vi "ProcessFMData.vi"(1 "Sensor Readings In":dbl[](array[numeric])) -> (0 "Sensor Readings Out":dbl[](array[numeric]))   [LabVIEW 2018]
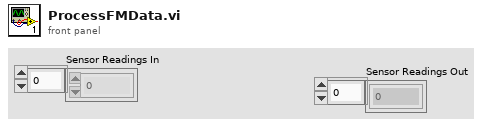
[diagram p1: front panel]
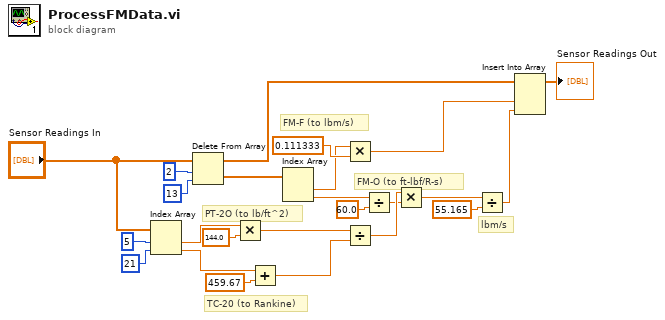
[diagram p0: block diagram]
diagram:
  # "FM-F (to lbm/s)"
  # "lbm/s"
  # "FM-O (to ft-lbf/R-s)"
  # "TC-20 (to Rankine)"
  # "PT-2O (to lb/ft^2)"
  n1 = Index Array(array="Sensor Readings In", index #1=5 ("index"), index #2=21 ("index")) -> (element #1=w15:dbl, element #2=w12:dbl)
  n2 = Delete From Array(array="Sensor Readings In", length=2, index=13) -> (deleted portion=w22:dbl[], array with subset deleted=w4:dbl[])
  n3 = Multiply(x=w15, y=144.0) -> (x*y=w10:dbl)
  n4 = Add(x=w12, y=459.67) -> (x+y=w9:dbl)
  n5 = Index Array(array=w22) -> (element #1=w20:dbl, element #2=w14:dbl)  [unwired: 2 in]
  n6 = Multiply(x=w20, y=0.111333) -> (x*y=w3:dbl)
  n7 = Divide(x=w10, y=w9) -> (x/y=w8:dbl)
  n8 = Divide(x=w14, y=60.0) -> (x/y=w7:dbl)
  n9 = Multiply(x=w8, y=w7) -> (x*y=w6:dbl)
  n10 = Divide(x=w6, y=55.165) -> (x/y=w2:dbl)
  n11 = Insert Into Array(array=w4, new element #1=w3, new element #2=w2) -> (→"Sensor Readings Out":dbl[])  [unwired: 1 in]
